vi "Manage Drive_1.vi"(7 "Min Drive Free Space (%)":dbl, 8 "error in":errorcluster, 11 "Data Folder":path=path "c:/data") -> (0 "error out":errorcluster, 2 "Drive Space Below Limit":bool, 3 "size (bytes)":i64)   [LabVIEW 2017]
panel:
  out "x*y":dbl
  out "free (bytes)":i64
  out "All Files in Dir":path[](array[path])
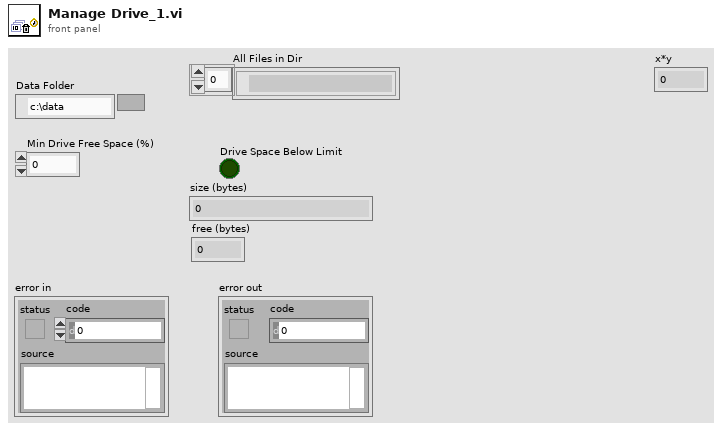
[diagram p1: front panel]
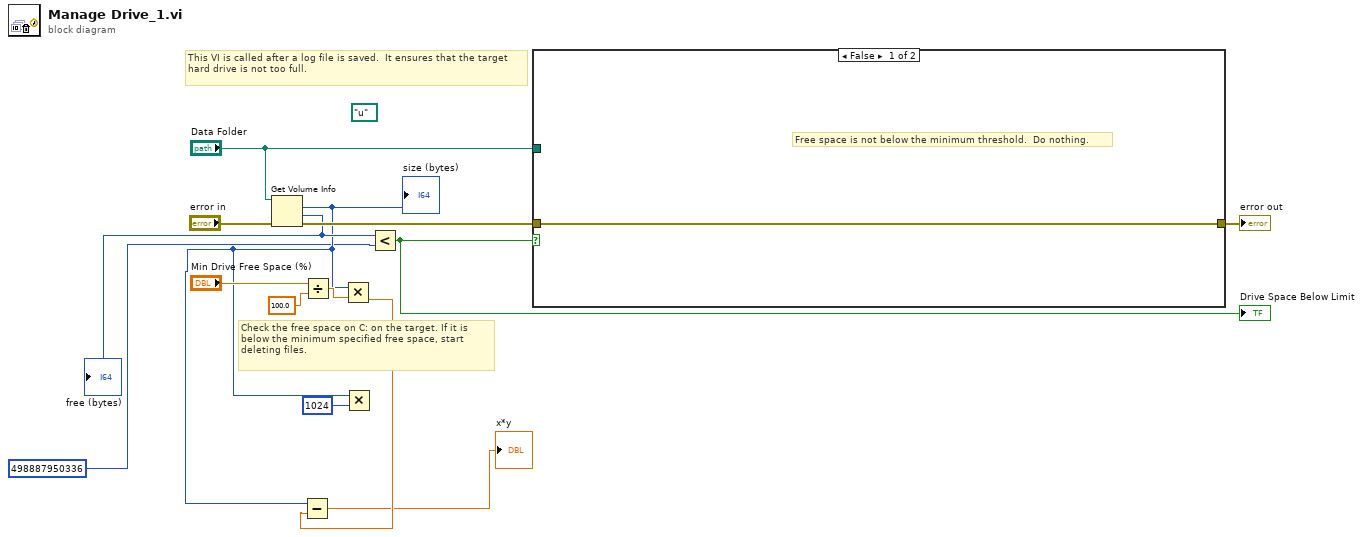
[diagram p0: block diagram]
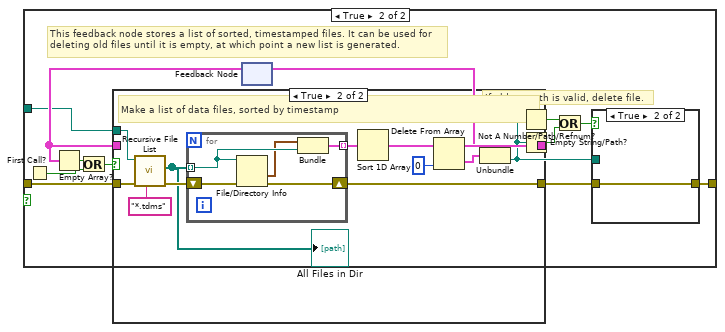
[diagram p2: hidden frame]
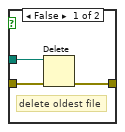
[diagram p3: hidden frame]
diagram:
  (unwired) path "u:/" ("AVI Path")
  # "Check the free space on C: on the target. If it is below the minimum specified free space, start deleting files."
  # "This VI is called after a log file is saved.  It ensures that the target hard drive is not too full."
  n1 = Get Volume Info(8:"error in", 11:"Data Folder") -> (0:w9:errorcluster, 1:w7:i64, 2:w4:i64)  [unwired: 3 out]
  "size (bytes)" <- w4
  "free (bytes)" <- w7
  n2 = Divide(x="Min Drive Free Space (%)", y=100.0) -> (x/y=w13:dbl)
  n3 = Multiply(x=w4, y=w13) -> (x*y=w3:dbl)
  n4 = Subtract(x=w4, y=w3) -> (x-y=→"x*y":dbl)
  n5 = Multiply(x=w4, y=i64 1024) -> ()  [unwired: 1 out]
  n6 = Less?(x=w7, y=i64 498887950336 ("free (bytes) 2")) -> (x < y?=w10:bool)
  "Drive Space Below Limit" <- w10
  n7 = case shown="False" w10 {
    tunnel: w9 -> [w15 w31]
    tunnel: [w15 w26] -> w8
    tunnel: "Data Folder" -> [_ w22]
    frame False {
      # "Free space is not below the minimum threshold.  Do nothing."
    }
    frame True {
      # "If oldest path is valid, delete file."
      # "This feedback node stores a list of sorted, timestamped files. It can be used for deleting old files until it is empty, at which point a new list is generated."
      n8 = First Call?() -> (First Call?: T/F=w29:bool)
      n9 = feedback #1() -> (w24:cluster{"last mod":timestamp, path}[])  [unwired: 1 out]
      n10 = Empty Array?(array=w24) -> (empty?=w23:bool)
      n11 = Or(x=w23, y=w29) -> (x .or. y?=w30:bool)
      n12 = case shown="True" w30 {
        tunnel: w31 -> [w37 w45]
        tunnel: [w37 w42] -> w25
        tunnel: [w36 w40] -> w28
        tunnel: w24 -> [w36 _]
        tunnel: w22 -> [_ w39]
        frame False {
          # "Current list of old files is non-empty.  Use it."
        }
        frame True {
          # "Make a list of data files, sorted by timestamp"
          n13 = call <vilib>:"Recursive File List.vi"("pattern"="*.tdms", "error in (no error)"=w45, "Folder Path"=w39) -> ("error out"=w43:errorcluster, "All Files in Dir"=w38:path[])  [unwired: 1 in, 6 out]
          "All Files in Dir" <- w38
          n14 = for {
            tunnel: w38 -> [w47] mode=indexing
            shift-right: [w49] -> w42
            shift-left: w43 -> [w50]
            tunnel: [w48] -> w41 mode=indexing
            n15 = File/Directory Info(path=w47, error in=w50) -> (last mod=w46:timestamp, error out=w49:errorcluster)  [unwired: 5 out]
            n16 = Bundle("last mod"=w46, w47) -> (w48:cluster{"last mod":timestamp, path})  [unwired: 1 out]
          }
          n17 = Sort 1D Array(array=w41) -> (sorted array=w40:cluster{"last mod":timestamp, path}[])
        }
      }
      n18 = Delete From Array(array=w28, index=0) -> (deleted portion=w20:cluster{"last mod":timestamp, path}, array with subset deleted=w27:cluster{"last mod":timestamp, path}[])  [unwired: 1 in]
      n19 = feedback-in #1(w27) -> ()
      n20 = Unbundle(w20) -> (w19:path)  [unwired: 1 out]
      n21 = Not A Number/Path/Refnum?(number/path/refnum=w19) -> (NaN/Path/Refnum?=w18:bool)
      n22 = Empty String/Path?(string/path=w19) -> (empty?=w17:bool)
      n23 = Or(x=w18, y=w17) -> (x .or. y?=w16:bool)
      n24 = case shown="True" w16 {
        tunnel: [w34 w35] -> w26
        tunnel: w25 -> [w33 w35]
        tunnel: w19 -> [w32 _]
        frame False {
          # "delete oldest file"
          n25 = Delete(path (use dialog)=w32, error in=w33) -> (error out=w34:errorcluster)  [unwired: 5 out]
        }
        frame True {
        }
      }
    }
  }
  "error out" <- w8
